vi "Unsub.vi"(8 "error in":errorcluster, 10 "NATS Client":refnum<class "NATS Client.lvclass">, 11 "NATS Subscription":refnum<class "NATS Subscription.lvclass">) -> (0 "error out":errorcluster, 3 "Unread Messages":T1[](array[typedef]))   [LabVIEW 2024, in "NATS Subscription.lvlib" / "NATS Subscription.lvclass"]
doc: "Unregisters a subscription with the client."
uses:
  NATS Subscription.lvclass
  NATS Client/NATS Client.lvclass
  <vilib>/NATS/NATS Core/Controls/nats message.ctl
  <vilib>/NATS/NATS Core/Controls/msg type.ctl
  NATS Subscription.lvclass/NATS Subscription.ctl
  get reply queue.vi
  <vilib>/NATS/NATS Core/NATS Core.lvlib
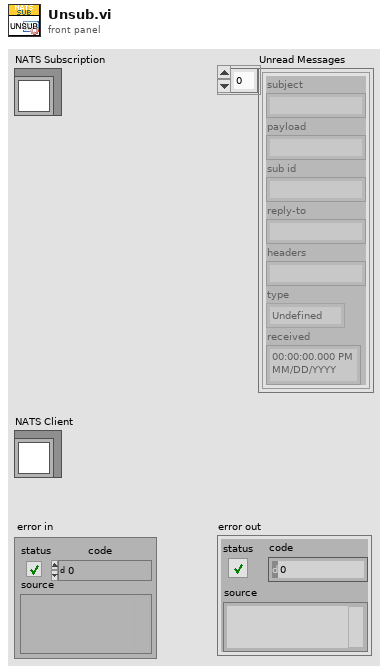
[diagram p1: front panel]
types:
  T1 = typedef "NATS Core.lvlib/nats message.ctl" = cluster{"subject":string, "payload":string, "sub id":string, "reply-to":string, "headers":string, "type":T2, "received":timestamp}
  T2 = typedef "NATS Core.lvlib/msg type.ctl" = enum16{"Undefined", "MSG", "HMSG", "+OK", "PING", "PONG", "-ERR", "INFO"}
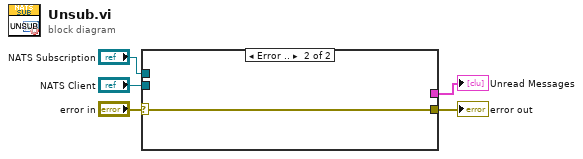
[diagram p0: block diagram]
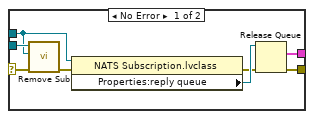
[diagram p2: hidden frame]
diagram:
  n1 = case shown="Error .." "error in" {
    selector: "error in" -> [w13 w14]
    tunnel: "NATS Client" -> [w12 _]
    tunnel: "NATS Subscription" -> [w11 _]
    tunnel: [w8 _] -> w2
    tunnel: [w7 w14] -> w1
    frame No Error {
      n2 = call "Remove Sub.vi"("error in"=w13, "NATS Subscription"=w11, "NATS Client in"=w12) -> ("error out"=w6:errorcluster)  [unwired: 7 in, 1 out]
      n3 = property class="NATS Subscription.lvclass"(reference=w11, error in=w6) -> (error out=w9:errorcluster, "Properties:reply queue"=w10:refnum<queue>)  [unwired: 1 out]
      n4 = Release Queue(queue=w10, error in (no error)=w9) -> (remaining elements=w8:T1[], error out=w7:errorcluster)  [unwired: 1 in, 1 out]
    }
    frame Error {
    }
  }
  "error out" <- w1
  "Unread Messages" <- w2
